vi "AMZ_S3_APIHLP_New Multipart Upload.vi"(8 "error in (no error)":errorcluster) -> (0 "error out":errorcluster, 3 "Multipart Upload RefNum":T1)   [LabVIEW 2015, in "LV Interface for Amazon S3.lvlib"]
uses:
  LV Interface for Amazon S3.lvlib
  Typedefs/AMZ_S3_Multipart Upload RefNum.ctl
  Typedefs/AMZ_S3_Multipart Upload RefNum Enum.ctl
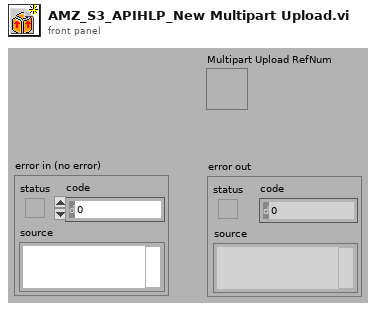
[diagram p1: front panel]
types:
  T1 = typedef "LV Interface for Amazon S3.lvlib/AMZ_S3_Multipart Upload RefNum.ctl" = refnum<k1>
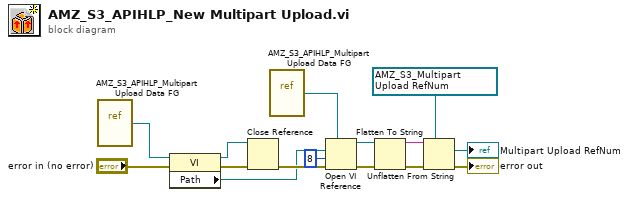
[diagram p0: block diagram]
diagram:
  w5 = T1 refnum items=["multipart upload"] ("Multipart Upload Reference")
  n1 = vi-ref "AMZ_S3_APIHLP_Multipart Upload Data FG.vi"() -> (w15:refnum<vi>)
  n2 = property class="VI"(reference=w15, error in="error in (no error)") -> (reference out=w13:refnum<vi>, error out=w14:errorcluster, "Path"=w11:path)
  n3 = Close Reference(reference=w13, error in (no error)=w14) -> (error out=w12:errorcluster)
  n4 = vi-ref "AMZ_S3_APIHLP_Multipart Upload Data FG.vi"() -> (w1:refnum<vi>)
  n5 = Open VI Reference(type specifier VI Refnum (for type only)=w1, vi path=w11, options=8, error in (no error)=w12) -> (vi reference=w7:refnum<vi>, error out=w8:errorcluster)  [unwired: 2 in]
  n6 = Flatten To String(anything=w7, error in (no error)=w8) -> (data string=w4:string, error out=w6:errorcluster)  [unwired: 2 in, 1 out]
  n7 = Unflatten From String(type=w5, binary string=w4, error in (no error)=w6) -> (value=→"Multipart Upload RefNum":T1, error out=→"error out":errorcluster)  [unwired: 2 in, 1 out]
